vi "DestroyClone.vi"(8 "error in (no error)":errorcluster, 9 "Exit via Stop Module Req?":bool, 10 "Wait for Module to stop?":bool, 11 "ModuleAdmin":refnum<class "ModuleAdmin.lvclass">) -> (0 "error out":errorcluster, 1 "External Launch":bool, 3 "Mod Admin out":refnum<class "ModuleAdmin.lvclass">)   [LabVIEW 2018, in "MyPlugins.lvlib"]
uses:
  MyPlugins/MyPlugins.lvlib
  <userlib>/NIST/ModuleAdminLib/ModuleAdmin/ModuleAdmin.lvclass
  C:/Program Files (x86)/National Instruments/LabVIEW 2018/user.lib/NIST/ModuleAdminLib/ModuleAdminBase/ModuleAdminBase.lvclass
  <userlib>/NIST/ModuleAdminLib/ModuleAdmin/ModuleAdmin.lvclass/ModuleAdmin.ctl
  <userlib>/NIST/ModuleAdminLib/ModuleAdmin/Accessors/Read CloneRegRef.vi
  <userlib>/NIST/ModuleAdminLib/CloneRegistration/CloneRegistration.lvclass
  MyPlugins/MyPluginBaseClass/MyPluginsBase.lvclass
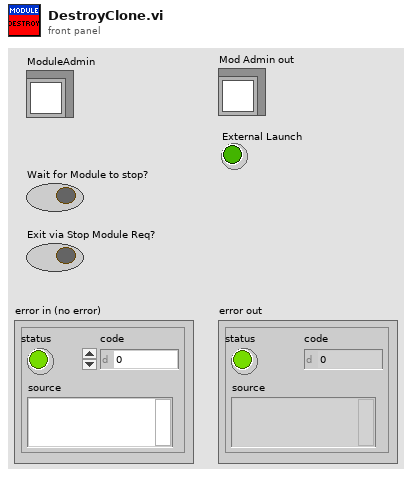
[diagram p1: front panel]
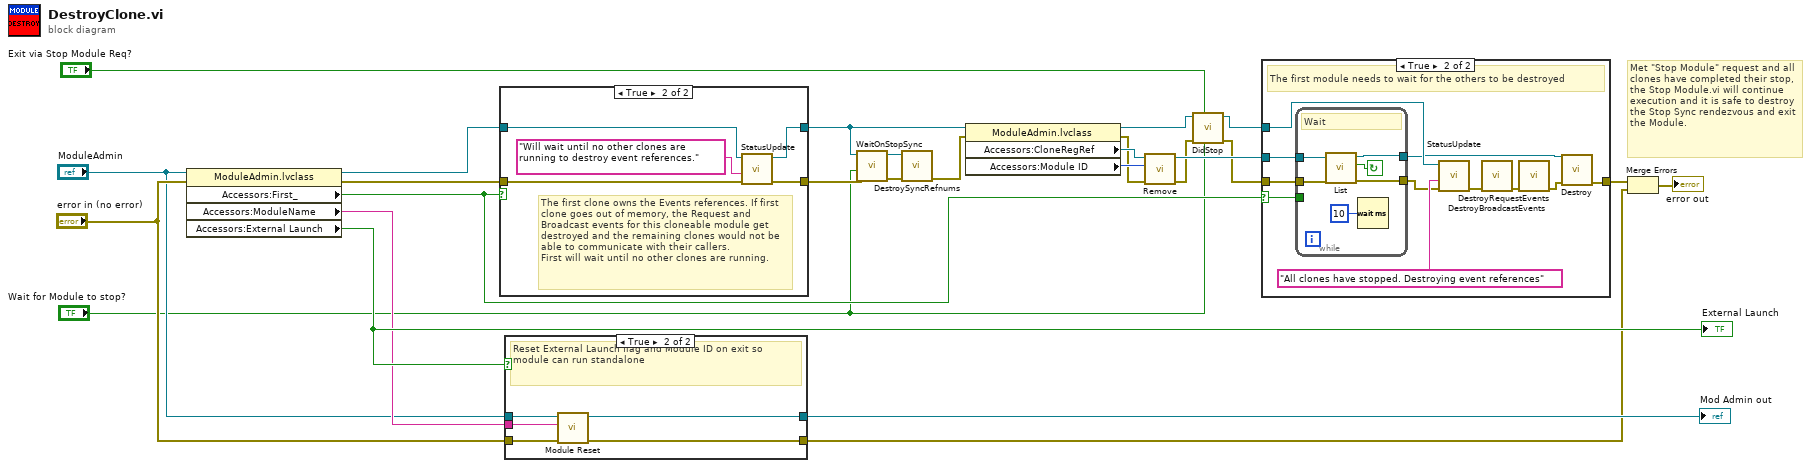
[diagram p0: block diagram]
diagram:
  # "Met \"Stop Module\" request and all clones have completed their stop, the Stop Module.vi will continue execution and it is safe to destroy the Stop Sync rendezvous and exit the Module."
  n1 = property class="ModuleAdmin.lvclass"(reference="ModuleAdmin", error in="error in (no error)") -> (reference out=w7:refnum<class "ModuleAdmin.lvclass">, error out=w8:errorcluster, "Accessors:First_"=w26:bool, "Accessors:ModuleName"=w22:string, "Accessors:External Launch"=w24:bool)
  "External Launch" <- w24
  n2 = case shown="True" w26 {
    tunnel: w8 -> [w28 w33]
    tunnel: [w28 w31] -> w12
    tunnel: w7 -> [w27 w30]
    tunnel: [w27 w29] -> w11
    frame False {
    }
    frame True {
      # "The first clone owns the Events references. If first clone goes out of memory, the Request and Broadcast events for this cloneable module get destroyed and the remaining clones would not be able to communicate with their callers.\nFirst will wait until no other clones are running."
      n3 = call "StatusUpdate.vi"("error in (no error)"=w33, "Status"="Will wait until no other clones are running to destroy event references." ("format string"), "Module"=w30) -> ("error out"=w31:errorcluster, "Module"=w29:refnum<class "ModuleAdmin.lvclass">)  [unwired: 7 in]
    }
  }
  n4 = case shown="True" w24 {
    tunnel: "error in (no error)" -> [w34 w40]
    tunnel: w22 -> [_ w39]
    tunnel: "ModuleAdmin" -> [w35 w38]
    tunnel: [w35 w37] -> w21
    tunnel: [w34 w36] -> w19
    frame False {
    }
    frame True {
      # "Reset External Launch flag and Module ID on exit so module can run standalone"
      n5 = call <userlib>:"Module Reset.vi"("error in (no error)"=w40, "ModuleName"=w39, "Mod Admin in"=w38) -> ("error out"=w36:errorcluster, "Mod Admin out"=w37:refnum<class "ModuleAdmin.lvclass">)  [unwired: 7 in]
    }
  }
  "Mod Admin out" <- w21
  n6 = call <userlib>:"WaitOnStopSync.vi"("error in (no error)"=w12, "WaitForModuleToStop?"="Wait for Module to stop?", "ModuleAdmin"=w11) -> ("error out"=w25:errorcluster, "ModuleAdmin"=w16:refnum<class "ModuleAdmin.lvclass">)  [unwired: 7 in]
  n7 = call <userlib>:"DestroySyncRefnums.vi"("error in (no error)"=w25, "ModuleAdmin"=w16) -> ("error out"=w10:errorcluster)  [unwired: 9 in]
  n8 = property class="ModuleAdmin.lvclass"(reference=w11, error in=w10) -> (reference out=w5:refnum<class "ModuleAdmin.lvclass">, error out=w9:errorcluster, "Accessors:CloneRegRef"=w15:refnum<data-value>, "Accessors:Module ID"=w14:i32)
  n9 = call <userlib>:"Remove.vi"("error in (no error)"=w9, "Module ID"=w14, "CloneRegRef"=w15) -> ("error out"=w3:errorcluster, "CloneRegRef"=w18:refnum<data-value>)  [unwired: 6 in, 1 out]
  n10 = call "DidStop.vi"("Wait for Module to stop?"="Wait for Module to stop?", "Exit via Stop Module Req?"="Exit via Stop Module Req?", "error in (no error)"=w3, "ModuleAdmin"=w5) -> ("error out"=w2:errorcluster, "ModuleAdmin"=w4:refnum<class "ModuleAdmin.lvclass">)  [unwired: 6 in]
  n11 = case shown="True" w26 {
    selector: w26 -> [_ w51]
    tunnel: w2 -> [w41 w52]
    tunnel: [w41 w44] -> w13
    tunnel: w18 -> [_ w46]
    tunnel: w4 -> [_ w45]
    frame False {
    }
    frame True {
      # "The first module needs to wait for the others to be destroyed"
      n12 = while {
        tunnel: w52 -> [w58]
        tunnel: w51 -> [_]
        tunnel: [w57] -> w49
        tunnel: w46 -> [w54]
        tunnel: [w53] -> w42
        stop <- w56 continue-if-true
        # "Wait"
        n13 = call <userlib>:"List.vi"("error in (no error)"=w58, "CloneRegRef"=w54) -> ("error out"=w57:errorcluster, "Found?"=w56:bool, "CloneRegRef"=w53:refnum<data-value>)  [unwired: 4 in, 3 out]
        n14 = Wait (ms)(milliseconds to wait=u32 10) -> ()  [unwired: 1 out]
      }
      n15 = call "StatusUpdate.vi"("error in (no error)"=w49, "Status"="All clones have stopped. Destroying event references", "Module"=w45) -> ("error out"=w48:errorcluster)  [unwired: 7 in, 1 out]
      n16 = call "DestroyBroadcastEvents.vi"("error in (no error)"=w48) -> ("error out"=w47:errorcluster)  [unwired: 10 in]
      n17 = call "DestroyRequestEvents.vi"("error in (no error)"=w47) -> ("error out"=w43:errorcluster)  [unwired: 10 in]
      n18 = call <userlib>:"Destroy.vi"("error in (no error)"=w43, "CloneRegRef"=w42) -> ("error out"=w44:errorcluster)  [unwired: 9 in]
    }
  }
  n19 = Merge Errors(w13, w19) -> (→"error out":errorcluster)
